vi "Set Temperature.vi"(8 "error in":errorcluster, 10 "Temperature":dbl, 11 "CnPt in":refnum<class "CnPt.lvclass">) -> (0 "error out":errorcluster, 3 "CnPt out":refnum<class "CnPt.lvclass">)   [LabVIEW 2015, in "CnPt.lvclass"]
uses:
  CnPt.lvclass
  <vilib>/MSR Consulting, LLC/General Reuse/Session APIs/Serial/Serial Session.lvclass
  CnPt.lvclass/CnPt.ctl
  <vilib>/MSR Consulting, LLC/General Reuse/Session APIs/Serial/Public/Asynchronous Write.vi
  <vilib>/MSR Consulting, LLC/General Reuse/Session APIs/Serial/Public/Asynchronous Read.vi
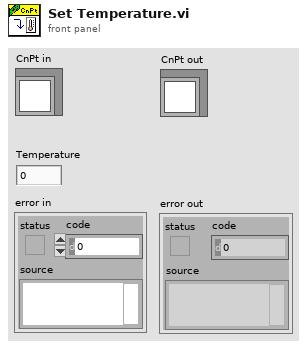
[diagram p1: front panel]
types:
  T1 = typedef "Serial Session.lvclass/Session Handle.ctl" = refnum<data-value>
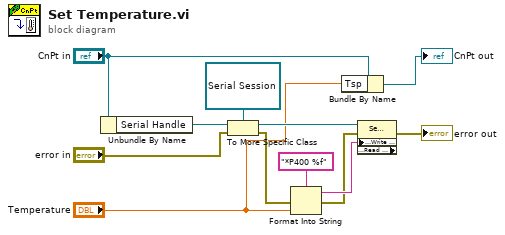
[diagram p0: block diagram]
diagram:
  n1 = Unbundle By Name("CnPt in") -> ("Serial Handle"=w12:T1)
  n2 = To More Specific Class(target class=refnum<data-value> refnum, reference=w12, error in="error in") -> (specific class reference=w10:refnum<data-value>, error out=w6:errorcluster)
  n3 = Format Into String(format string="*P400 %f", error in=w6, "Temperature") -> (resulting string=w8:string, error out=w5:errorcluster)  [unwired: 1 in]
  n4 = Bundle By Name(cluster="CnPt in", "Tsp"="Temperature") -> (→"CnPt out":refnum<class "CnPt.lvclass">)
  n5 = property class="Serial Session" props=["Public:Write - Asynchronous", "Public:Read - Asynchronous"](reference=w10, error in=w5, "Public:Write - Asynchronous"=w8) -> (error out=→"error out":errorcluster)  [unwired: 2 out]
